vi "Echo.vi"(8 "error in (no error)":errorcluster, 11 "VISA resource name":refnum<visa-resource-name>) -> (0 "error out":errorcluster, 2 "ECHO":bool, 3 "VISA resource name out":refnum<visa-resource-name>)   [LabVIEW 2017, in "Spectral Products CM110.lvlib"]
uses:
  Spectral Products CM110.lvlib
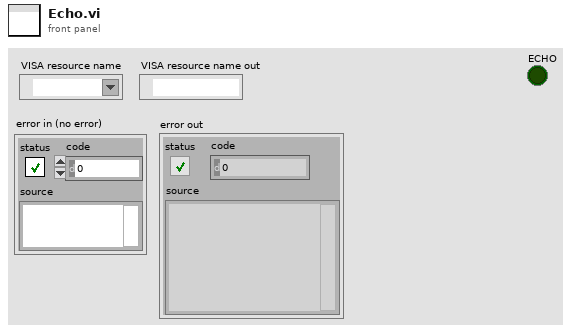
[diagram p1: front panel]
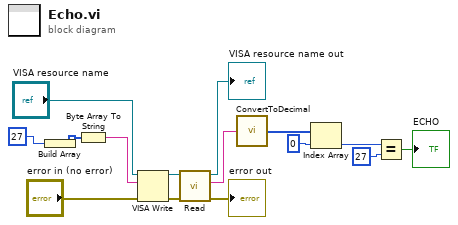
[diagram p0: block diagram]
diagram:
  n1 = Build Array(u8 27) -> (w2:u8[])
  n2 = Byte Array To String(unsigned byte array=w2) -> (string=w1:string)
  n3 = VISA Write(VISA resource name="VISA resource name", write buffer=w1, error in (no error)="error in (no error)") -> (VISA resource name out=w14:refnum<visa-resource-name>, error out=w15:errorcluster)  [unwired: 1 out]
  n4 = call "Read.vi"("error in (no error)"=w15, "VISA Refnum in"=w14) -> ("error out"=→"error out":errorcluster, "read buffer"=w9:string, "VISA Refnum out"=→"VISA resource name out":refnum<visa-resource-name>)  [unwired: 6 in, 1 out]
  n5 = call "ConvertToDecimal.vi"("read buffer"=w9) -> ("unsigned byte array"=w8:u8[])
  n6 = Index Array(array=w8, index=0) -> (element=w6:u8)
  n7 = Equal?(x=w6, y=27) -> (x = y?=→"ECHO":bool)
